vi "read_environment (SubVI).vi"(10 "Read pressures?":bool, 11 "Read temps?":bool) -> (3 "Temp array":dbl[](array[numeric]))   [LabVIEW 2014]
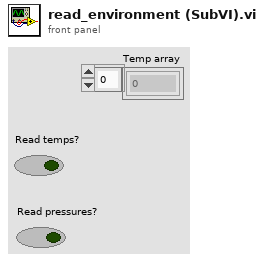
[diagram p1: front panel]
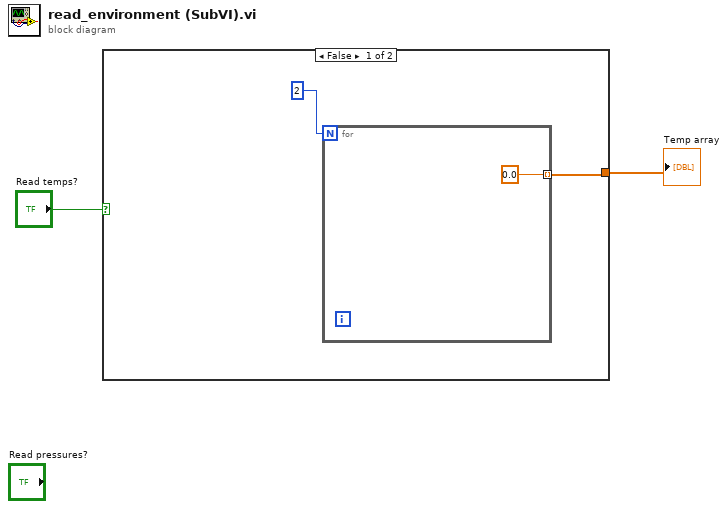
[diagram p0: block diagram]
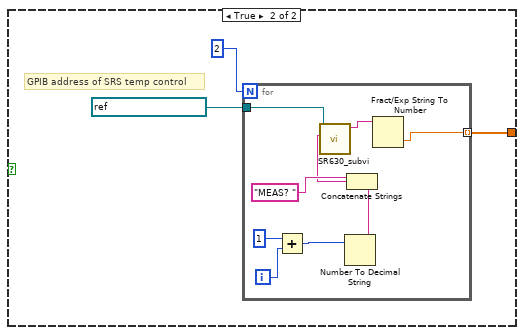
[diagram p2: hidden frame]
diagram:
  n1 = case shown="False" "Read temps?" {
    tunnel: [w3 w6] -> w2
    frame False {
      n2 = for {
        N: 2 ("dimension size") -> [_]
        tunnel: [0.0] -> w3 mode=indexing
      }
    }
    frame True {
      # "GPIB address of SRS temp control"
      n3 = for {
        N: 2 ("dimension size") -> [_]
        tunnel: refnum<visa-resource-name> "GPIB0::19::INSTR" ("VISA Refnum in") -> [w17]
        tunnel: [w15] -> w6 mode=indexing
        i -> [w14]
        n4 = Add(x=1, y=w14) -> (x+y=w12:i32)
        n5 = Number To Decimal String(number=w12) -> (decimal integer string=w11:string)  [unwired: 1 in]
        n6 = Concatenate Strings("MEAS? " ("Write Buffer"), w11) -> (w9:string)
        n7 = call "SR630_subvi.vi"("Write Buffer"=w9, "VISA Refnum in"=w17) -> ("read buffer"=w16:string)  [unwired: 9 in]
        n8 = Fract/Exp String To Number(string=w16) -> (number=w15:dbl)  [unwired: 3 in, 1 out]
      }
    }
  }
  "Temp array" <- w2
